vi "Validate Initial State.vi"(8 "error in":errorcluster, 9 "initial state":string, 10 "state names":string[](array[string])) -> (0 "error out":errorcluster, 2 "index found":i32)   [LabVIEW 2020, in "Routing and Faulting Scripting.lvlib"]
uses:
  Routing and Faulting Scripting.lvlib
  <vilib>/Utility/error.llb/Error Cluster From Error Code.vi
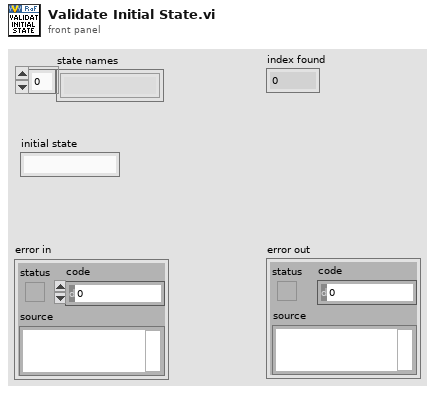
[diagram p1: front panel]
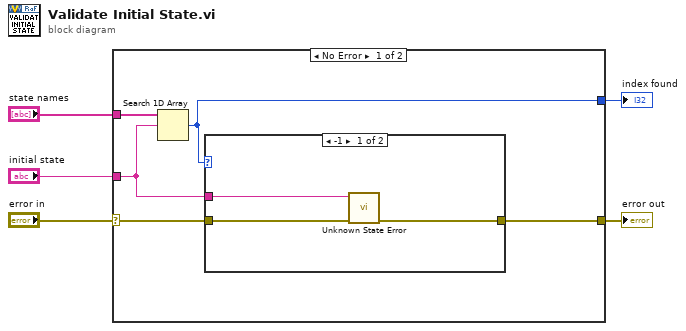
[diagram p0: block diagram]
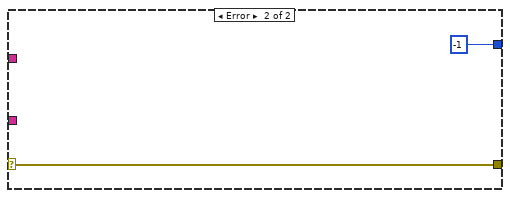
[diagram p3: hidden frame]
diagram:
  n1 = case shown="No Error" "error in" {
    selector: "error in" -> [w10 w16]
    tunnel: [w9 w16] -> w4
    tunnel: "state names" -> [w8 _]
    tunnel: "initial state" -> [w6 _]
    tunnel: [w7 -1 ("index of element")] -> w1
    frame No Error {
      n2 = Search 1D Array(1D array=w8, element=w6) -> (index of element=w7:i32)  [unwired: 1 in]
      n3 = case shown="-1" w7 {
        tunnel: w10 -> [w13 w14]
        tunnel: [w12 w14] -> w9
        tunnel: w6 -> [w11 _]
        frame -1 {
          n4 = call "Unknown State Error.vi"("error in (no error)"=w13, "state"=w11) -> ("error out"=w12:errorcluster)  [unwired: 9 in]
        }
        frame Default {
        }
      }
    }
    frame Error {
    }
  }
  "error out" <- w4
  "index found" <- w1
